vi "Read Key Boolean.vi"(6 "Default Val":bool, 7 "Section Name":string, 8 "error in (no error)":errorcluster, 10 "Key Names":string, 11 "Config Data":T1(array[cluster])) -> (0 "error out":errorcluster, 1 "Key Names":string[](array[string]), 2 "Key Value out":bool, 3 "Config Data dup":T1(array[cluster]), 4 "Key Find?":bool)   [LabVIEW 2020, in "GUCalibration2.lvlib"]
uses:
  GUCalibration2.lvlib
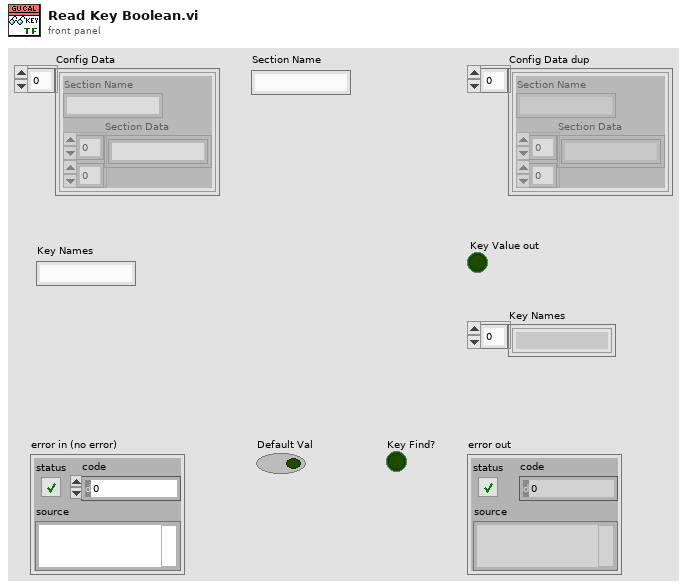
[diagram p1: front panel]
types:
  T1 = cluster{"Section Name":string, "Section Data":string[][]}[]
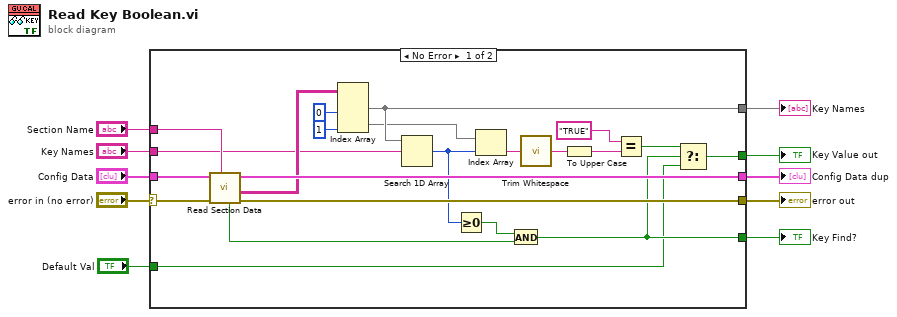
[diagram p0: block diagram]
diagram:
  n1 = case shown="No Error" "error in (no error)" {
    selector: "error in (no error)" -> [w30 w34]
    tunnel: "Section Name" -> [w31 _]
    tunnel: "Config Data" -> [w32 w33]
    tunnel: [w24 w34] -> w7
    tunnel: [w29 w33] -> w6
    tunnel: [w26 _] -> w5
    tunnel: "Key Names" -> [w25 _]
    tunnel: [w18 _] -> w3
    tunnel: "Default Val" -> [w17 _]
    tunnel: [w16 _] -> w1
    frame No Error {
      n2 = call "Read Section Data.vi"("Section Name"=w31, "error in (no error)"=w30, "Config Data"=w32) -> ("error out"=w24:errorcluster, "Section Data"=w28:string[][], "Config Data out"=w29:T1, "Section Exist"=w19:bool)  [unwired: 4 in, 1 out]
      n3 = Index Array(array=w28, index (col) #1=0 ("disabled index (col)"), index (col) #2=1 ("index (col)")) -> (element #1=w26:string[], element #2=w22:string[])  [unwired: 2 in]
      n4 = Search 1D Array(1D array=w26, element=w25) -> (index of element=w21:i32)  [unwired: 1 in]
      n5 = Greater Or Equal To 0?(x=w21) -> (x >= 0?=w20:bool)
      n6 = Index Array(array=w22, index=w21) -> (element=w15:string)
      n7 = And(x=w20, y=w19) -> (x .and. y?=w18:bool)
      n8 = call <vilib>:"Trim Whitespace.vi"("string"=w15) -> ("trimmed string"=w14:string)  [unwired: 1 in]
      n9 = To Upper Case(1:w14) -> (0:w13:string)
      n10 = Equal?(x="TRUE", y=w13) -> (x = y?=w11:bool)
      n11 = Select(t=w11, s=w18, f=w17) -> (s? t:f=w16:bool)
    }
    frame Error {
    }
  }
  "error out" <- w7
  "Key Names" <- w5
  "Config Data dup" <- w6
  "Key Find?" <- w3
  "Key Value out" <- w1
